vi "Analog DC Generation.vi"(0 "RegenMode":i32(ring)=10097 items=["Allow Regeneration"=10097, "Do Not Allow Regeneration"=10158], 1 "SampTimingType":i32(ring)=10388 items=["Sample Clock"=10388, "Burst Handshake"=12548, "Handshake"=10389, "Implicit"=10451, "On Demand"=10390, "Change Detection"=12504, "Pipelined Sample Clock"=14668], 2 "output terminal configuration":i32(ring)=-1 items=["Default"=-1, "RSE"=10083, "Differential"=10106, "Pseudodifferential"=12529], 3 "physical channels":tag, 4 "data":dbl format="%0.2f") -> (5 "error out":errorcluster)   [LabVIEW 2019, in "SubVIs.lvlib" / "Torque VI.lvlib"]
uses:
  <vilib>/DAQmx/write.llb/DAQmx Write (Analog DBL 1Chan 1Samp).vi
  <vilib>/DAQmx/create/channels.llb/DAQmx Create Channel (AO-Voltage-Basic).vi
  <vilib>/DAQmx/miscellaneous.llb/DAQmx Fill In Error Info.vi
  Torque VI.lvlib
  <resource>/objmgr/daqmx.rc
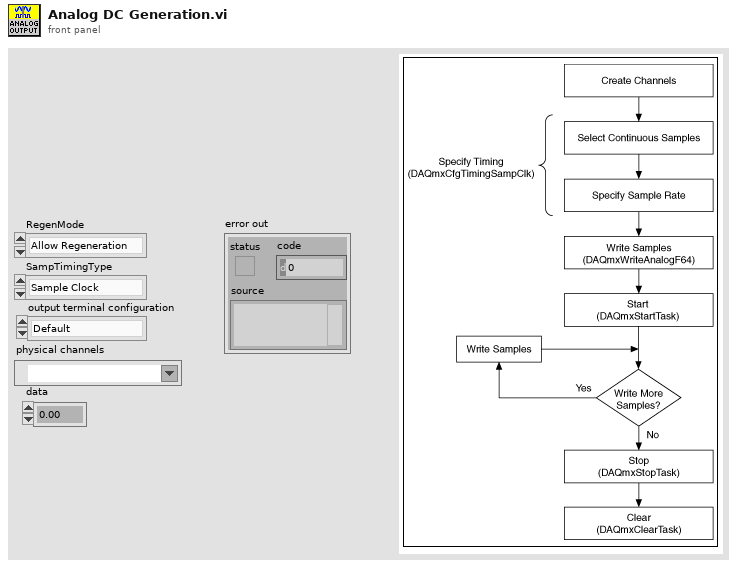
[diagram p1: front panel]
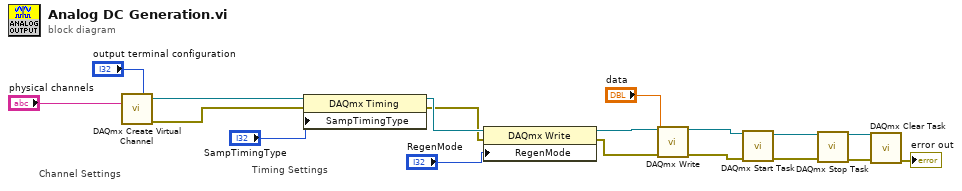
[diagram p0: block diagram]
diagram:
  # "Timing Settings"
  # "Channel Settings"
  n1 = call-poly <vilib>:"DAQmx Create Virtual Channel.vi"("output terminal configuration"="output terminal configuration", "physical channels"="physical channels") -> ("task out"=w18:refnum<k21>, "error out"=w17:errorcluster)  [unwired: 12 in]
  n2 = property class="DAQmx Timing"(reference=w18, error in=w17, "SampTimingType"="SampTimingType") -> (reference out=w14:refnum<k21>, error out=w13:errorcluster)
  n3 = property class="DAQmx Write"(reference=w14, error in=w13, "RegenMode"="RegenMode") -> (reference out=w12:refnum<k21>, error out=w11:errorcluster)
  n4 = call-poly <vilib>:"DAQmx Write.vi"("task/channels in"=w12, "data"="data", "error in"=w11) -> ("task out"=w16:refnum<k21>, "error out"=w15:errorcluster)  [unwired: 10 in, 1 out]
  n5 = call <vilib>:"DAQmx Start Task.vi"("task/channels in"=w16, "error in"=w15) -> ("task out"=w2:refnum<k21>, "error out"=w3:errorcluster)  [unwired: 12 in]
  n6 = call <vilib>:"DAQmx Stop Task.vi"("task/channels in"=w2, "error in"=w3) -> ("task out"=w4:refnum<k21>, "error out"=w5:errorcluster)  [unwired: 12 in]
  n7 = call <vilib>:"DAQmx Clear Task.vi"("task in"=w4, "error in"=w5) -> ("error out"=→"error out":errorcluster)  [unwired: 13 in]
